vi "Get Directly Owned Objects.vi"(1 "Top Object":refnum<vi>, 2 "Nested Objects":refnum<vi>[](array[refnum])) -> (0 "Directly Owned Objects":refnum<vi>[](array[refnum]))   [LabVIEW 2014]
doc: "Returns objects which are directly owned by specified object. So if there's wired i.e. WhileLoop and references of loopTunnel, it erase LoopTunnel which are located at nested WhileLoop."
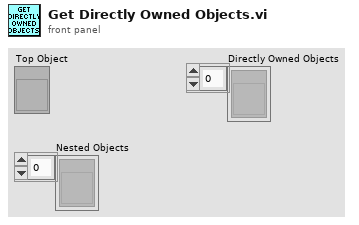
[diagram p1: front panel]
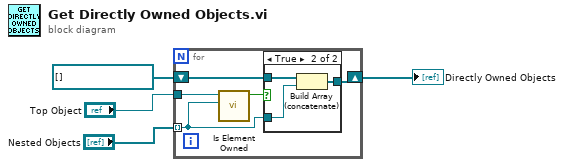
[diagram p0: block diagram]
diagram:
  n1 = for {
    tunnel: "Nested Objects" -> [w8] mode=indexing
    shift-right: [w7] -> w3
    shift-left: refnum<vi>[] [] -> [w6]
    tunnel: "Top Object" -> [w5]
    n2 = call "Is Element Owned.vi"("Nested Object"=w8, "Relative Object"=w5) -> ("is owned?"=w9:bool)  [unwired: 9 in]
    n3 = case shown="True" w9 {
      tunnel: w8 -> [_ w13]
      tunnel: [w10 w12] -> w7
      tunnel: w6 -> [w10 w11]
      frame False {
      }
      frame True {
        n4 = Build Array (concatenate)(w11, w13) -> (w12:refnum<vi>[])
      }
    }
  }
  "Directly Owned Objects" <- w3
